vi "DSP Reset Control.vi"(1 "reset in":bool, 2 "mask 1":bool, 3 "mask 2":bool, 4 "ready for input":bool[](array[boolean])) -> (15 "reset out":bool, 16 "masked 1 reset out":bool, 17 "masked 2 reset out":bool, 18 "reset done":bool)   [LabVIEW 2018, in "GettingStarted_5774_FPGA.lvlib"]
doc: "Provides the DSP chain reset signal and monitors the reset completion.\n\nThe <B>reset in</B> input is the DSP chain reset request input. The <B>reset out</B> output returns the <B>reset in</B> input with 2 clock cycles delay, the <B>masked 1 reset out</B> output returns the logic AND of the <B>reset in</B> and <B>mask 1</B> inputs with 2 clock cycles delay, while the <B>masked 2 reset out</B> output returns the logic AND of the <B>reset in</B> and <B>mask 2</B> inputs with 2 clock cycles delay. Connect the <B>reset out</B>, the <B>masked 1 reset out</B> or the <B>masked 2 reset out</B> outputs to the reset input of the DSP blocks.\n\nThe <B>ready for input</B> is an array of booleans for receiving the ready for input signals from the DSP blocks. These signals are used to detect the reset completion of the DSP blocks. Connect the ready for input outputs of the DSP blocks to this input through a (Build Array and a) Feedback Node.\n\nThe <B>reset done</B> output signals the DSP chain reset completion. A true on the <B>reset in</B> input sets this output to false. This output becomes (and remains) true if all elements of the <B>ready for input</B> array is true."
uses:
  <instrlib>/_niInstr/Basic Elements/v1/FPGA/Public/Max Fanout.ctl
  <instrlib>/_niInstr/Basic Elements/v1/FPGA/Private/Count Down U8.vi
  GettingStarted_5774_FPGA.lvlib
  <instrlib>/_niInstr/Basic Elements/v1/FPGA/niInstr Basic Elements v1 FPGA.lvlib
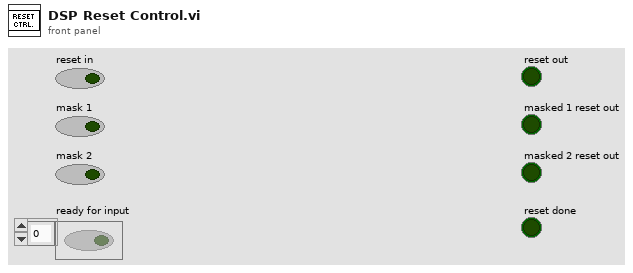
[diagram p1: front panel]
types:
  T1 = typedef "niInstr Basic Elements v1 FPGA.lvlib/Max Fanout.ctl" = enum16{"4", "8", "16", "32"}
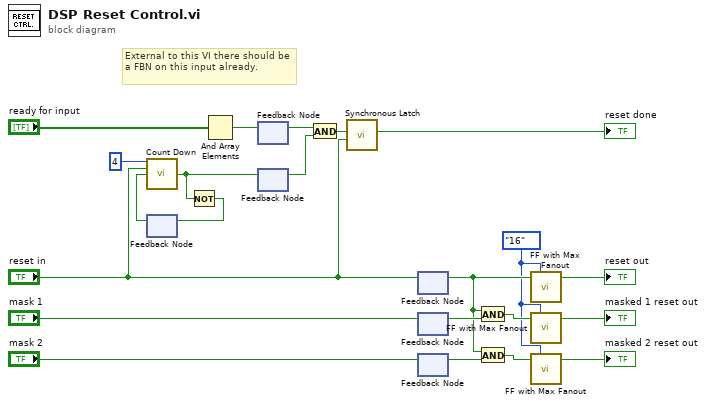
[diagram p0: block diagram]
diagram:
  w2 = Max_Fanout."16" ("kMaxFanout")
  # "External to this VI there should be a FBN on this input already."
  n1 = feedback #1() -> (w15:bool)  [unwired: 1 in]
  n2 = call-poly <instrlib>:"Count Down.vi"("count in"=u8 4, "load"="reset in", "decrement"=w15) -> ("terminal count"=w14:bool)  [unwired: 11 in, 1 out]
  n3 = Not(x=w14) -> (.not. x?=w16:bool)
  n4 = feedback-in #1(w16) -> ()
  n5 = And Array Elements(Boolean array="ready for input") -> (logical AND=w18:bool)
  n6 = feedback-in #2(w18) -> ()
  n7 = feedback #2() -> (w13:bool)  [unwired: 1 in]
  n8 = feedback #3() -> (w12:bool)  [unwired: 1 in]
  n9 = feedback-in #3(w14) -> ()
  n10 = And(x=w13, y=w12) -> (x .and. y?=w11:bool)
  n11 = call <instrlib>:"Synchronous Latch.vi"("clear"="reset in", "set"=w11) -> ("out"=→"reset done":bool)  [unwired: 9 in]
  n12 = feedback-in #4("reset in") -> ()
  n13 = feedback #4() -> (w4:bool)  [unwired: 1 in]
  n14 = feedback #5() -> (w22:bool)  [unwired: 1 in]
  n15 = feedback-in #5("mask 1") -> ()
  n16 = feedback #6() -> (w5:bool)  [unwired: 1 in]
  n17 = feedback-in #6("mask 2") -> ()
  n18 = And(x=w4, y=w22) -> (x .and. y?=w20:bool)
  n19 = And(x=w4, y=w5) -> (x .and. y?=w3:bool)
  n20 = call <instrlib>:"FF with Max Fanout.vi"("cDataIn"=w4, "kMaxFanout"=w2) -> ("cDataOut"=→"reset out":bool)  [unwired: 13 in]
  n21 = call <instrlib>:"FF with Max Fanout.vi"("cDataIn"=w20, "kMaxFanout"=w2) -> ("cDataOut"=→"masked 1 reset out":bool)  [unwired: 13 in]
  n22 = call <instrlib>:"FF with Max Fanout.vi"("cDataIn"=w3, "kMaxFanout"=w2) -> ("cDataOut"=→"masked 2 reset out":bool)  [unwired: 13 in]
